vi "Start-Stop DAQ.vi"(8 "Error In":errorcluster, 10 "Start DAQ":bool, 11 "LHW-Aquisition-Actor in":refnum<class "LHW-Aquisition-Actor.lvclass">) -> (0 "Error Out":errorcluster, 3 "LHW-Aquisition-Actor out":refnum<class "LHW-Aquisition-Actor.lvclass">)   [LabVIEW 2016, in "LHW-Acquisition.lvlib" / "LHW-Aquisition-Actor.lvclass"]
doc: "Start/Stop DAQ and update called DAQ Active status."
uses:
  LHW-Aquisition-Actor.lvclass
  C:/Program Files (x86)/National Instruments/LabVIEW 2016/vi.lib/ActorFramework/Actor/Actor.lvclass
  <vilib>/ActorFramework/Actor/Actor.lvclass/Actor.ctl
  <vilib>/ActorFramework/Time-Delayed Send Message/Time-Delay Override Options.ctl
  LHW-Aquisition-Actor.lvclass/LHW-Aquisition-Actor.ctl
  LHW-Aquisition-Actor Messages/Acquire Data Msg/Acquire Data Msg.lvclass
  C:/Program Files (x86)/National Instruments/LabVIEW 2016/vi.lib/ActorFramework/Message/Message.lvclass
  <vilib>/ActorFramework/Message Enqueuer/Message Enqueuer.lvclass/Message Enqueuer.ctl
  LHW-GUI-Actor Messages/Update DAQ Active Msg/Update DAQ Active Msg.lvclass/Update DAQ Active Msg.ctl
  <vilib>/ActorFramework/Message Enqueuer/Init from Existing Queue.vi
  <vilib>/ActorFramework/Message Enqueuer/Enqueue.vi
  LHW-GUI-Actor Messages/Update DAQ Active Msg/Update DAQ Active Msg.lvclass
  <vilib>/ActorFramework/Message Priority Queue/Priority Enqueue.vi
  <vilib>/ActorFramework/Message Enqueuer/Message Enqueuer.lvclass
  <vilib>/ActorFramework/Actor/Actor.lvclass
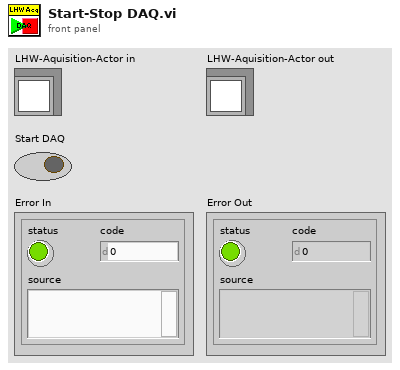
[diagram p1: front panel]
types:
  T1 = typedef "Time-Delay Override Options.ctl" = enum16{"Send next copy now", "Skip next scheduled copy", "Send next copy now and stop all further copies", "Stop all further copies"}
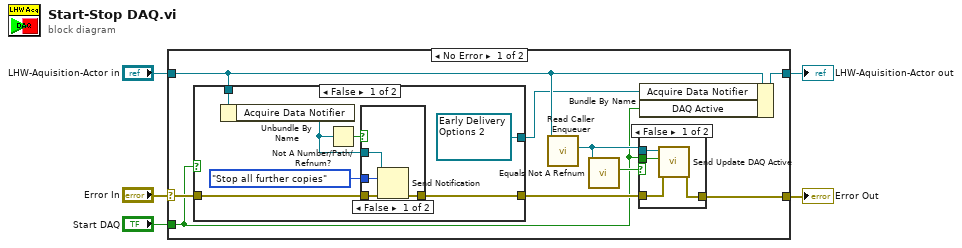
[diagram p0: block diagram]
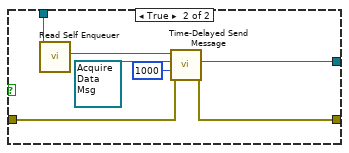
[diagram p3: hidden frame]
diagram:
  n1 = case shown="No Error" "Error In" {
    selector: "Error In" -> [w9 w40]
    tunnel: [w13 w40] -> w4
    tunnel: [w14 w39] -> w2
    tunnel: "LHW-Aquisition-Actor in" -> [w10 w39]
    tunnel: "Start DAQ" -> [w6 _]
    frame No Error {
      n2 = case shown="False" w6 {
        tunnel: w10 -> [w21 w33]
        tunnel: w9 -> [w19 w31]
        tunnel: [w18 w30] -> w8
        tunnel: [w17 w27] -> w7
        frame False {
          w17 = refnum<notifier> refnum items=["Send next copy now", "Skip next scheduled copy", "Send next copy now and stop all further copies", "Stop all further copies"] ("Delivery Notifier")
          n3 = Unbundle By Name(w21) -> ("Acquire Data Notifier"=w15:refnum<notifier>)
          n4 = Not A Number/Path/Refnum?(number/path/refnum=w15) -> (NaN/Path/Refnum?=w16:bool)
          n5 = case shown="False" w16 {
            tunnel: w15 -> [w25 _]
            tunnel: Time-Delay_Override_Options."Stop all further copies" ("notification") -> [w24 _]
            tunnel: w19 -> [w23 w26]
            tunnel: [w22 w26] -> w18
            frame False {
              n6 = Send Notification(notification=w24, notifier=w25, error in (no error)=w23) -> (error out=w22:errorcluster)  [unwired: 1 out]
            }
            frame True {
            }
          }
        }
        frame True {
          n7 = call <vilib>:"Read Self Enqueuer.vi"("Actor"=w33) -> ("Self Enqueuer"=w32:refnum<class "Message Enqueuer.lvclass">)  [unwired: 10 in]
          n8 = call <vilib>:"Time-Delayed Send Message.vi"("error in (no error)"=w31, "Milliseconds To Wait"=1000, "Message"=refnum<class "Acquire Data Msg.lvclass"> refnum ("LHW-Acquisition.lvlib:Acquire Data Msg.lvclass"), "Message Enqueuer"=w32) -> ("error out"=w30:errorcluster, "Delivery Notifier"=w27:refnum<notifier>)  [unwired: 6 in]
        }
      }
      n9 = call <vilib>:"Read Caller Enqueuer.vi"("Actor"=w10) -> ("Caller Enqueuer"=w12:refnum<class "Message Enqueuer.lvclass">)  [unwired: 10 in]
      n10 = call <vilib>:"Equals Not A Refnum.vi"("Message Enqueuer"=w12) -> ("Not a refnum?"=w11:bool)  [unwired: 10 in]
      n11 = case shown="False" w11 {
        tunnel: w6 -> [w37 _]
        tunnel: w8 -> [w36 w38]
        tunnel: [w35 w38] -> w13
        tunnel: w12 -> [w34 _]
        frame False {
          n12 = call "Send Update DAQ Active.vi"("error in (no error)"=w36, "DAQ Active"=w37, "Message Enqueuer"=w34) -> ("error out"=w35:errorcluster)  [unwired: 7 in, 1 out]
        }
        frame True {
        }
      }
      n13 = Bundle By Name(cluster=w10, "Acquire Data Notifier"=w7, "DAQ Active"=w6) -> (w14:refnum<class "LHW-Aquisition-Actor.lvclass">)
    }
    frame Error {
    }
  }
  "Error Out" <- w4
  "LHW-Aquisition-Actor out" <- w2
